vi "CALC_Length_of_True_state_(in_time).vi"(2 "Frame timestamp":timestamp format="%<%x %.3X>T", 3 "Reset? (F)":bool, 4 "True state input":bool) -> (1 "True was kept for, s":dbl)   [LabVIEW 2018, in "Tracker.lvlib"]
uses:
  Tracker.lvlib
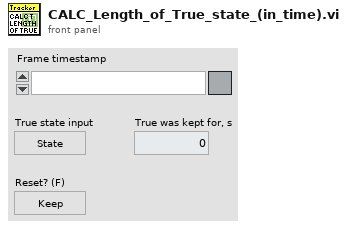
[diagram p1: front panel]
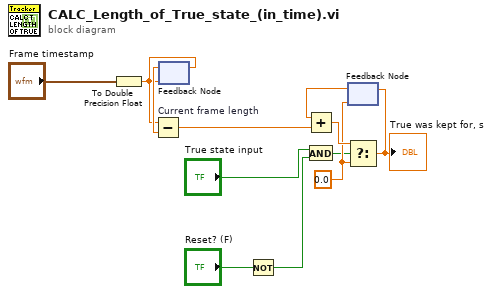
[diagram p0: block diagram]
diagram:
  w4 = 0.0 ("t")
  n1 = To Double Precision Float(number="Frame timestamp") -> (double precision float=w10:dbl)
  n2 = feedback-in #1(w10) -> ()
  n3 = feedback #1(w10) -> (w11:dbl)
  n4 = Subtract "Current frame length"(x=w10, y=w11) -> (x-y=w9:dbl)
  n5 = Not(x="Reset? (F)") -> (.not. x?=w1:bool)
  n6 = And(x="True state input", y=w1) -> (x .and. y?=w3:bool)
  n7 = feedback #2(w4) -> (w7:dbl)
  n8 = Add(x=w7, y=w9) -> (x+y=w5:dbl)
  n9 = Select(t=w5, s=w3, f=w4) -> (s? t:f=w8:dbl)
  "True was kept for, s" <- w8
  n10 = feedback-in #2(w8) -> ()
